vi "ActionVIOnDownload.vi"(5 "System Definition Dir":path, 6 "IP address":string, 7 "Details Ref":refnum<vi>, 8 "error in (no error)":errorcluster, 10 "WebDAV session in":T1, 11 "Device Item Ref in":T2 format="%.0x") -> (0 "error out":errorcluster, 2 "WebDAV session out":T1, 3 "Device Item Ref out":T2 format="%.0x")   [LabVIEW 2020, in "XNET System Explorer.lvlib"]
uses:
  XNET System Explorer.lvlib
  <vilib>/NI VeriStand/Custom Device API/Custom Device Item Ref.ctl
  <vilib>/WebDAVClient/Advanced/SessionHandle.ctl
  Includes/XNET System Explorer.lvlibp/System Explorer/Implementation/Implementation.lvlib
  <vilib>/NI VeriStand/Custom Device API/Custom Device API.lvlib
  <vilib>/WebDAVClient/NI_WebDAV.lvlib
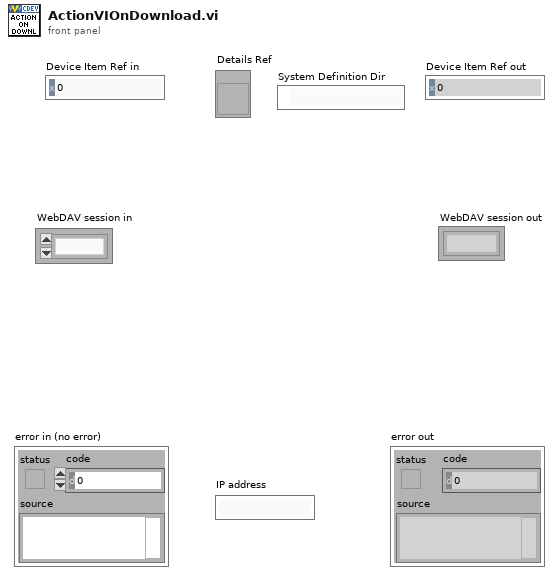
[diagram p1: front panel]
types:
  T1 = typedef "NI_WebDAV.lvlib/SessionHandle.ctl" = refnum<k1>
  T2 = typedef "Custom Device API.lvlib/Custom Device Item Ref.ctl" = u64
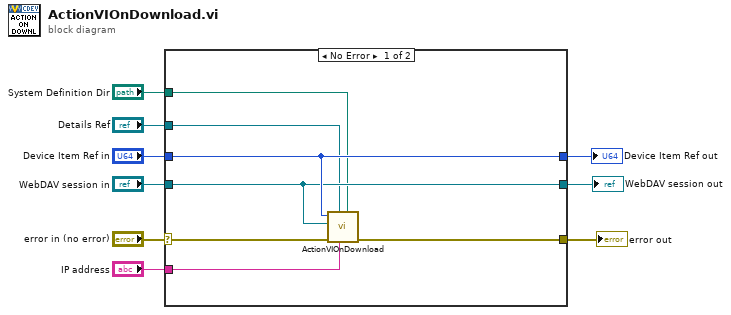
[diagram p0: block diagram]
diagram:
  n1 = case shown="No Error" "error in (no error)" {
    selector: "error in (no error)" -> [w16 w19]
    tunnel: [w15 w19] -> w8
    tunnel: "WebDAV session in" -> [w13 w18]
    tunnel: [w13 w18] -> w4
    tunnel: "Device Item Ref in" -> [w14 w17]
    tunnel: [w14 w17] -> w6
    tunnel: "Details Ref" -> [w12 _]
    tunnel: "IP address" -> [w11 _]
    tunnel: "System Definition Dir" -> [w10 _]
    frame No Error {
      n2 = call "ActionVIOnDownload.vi"("System Definition Dir"=w10, "IP address"=w11, "Details Ref"=w12, "error in (no error)"=w16, "WebDAV session in"=w13, "Device Item Ref in"=w14) -> ("error out"=w15:errorcluster)  [unwired: 3 in, 2 out]
    }
    frame Error {
    }
  }
  "error out" <- w8
  "Device Item Ref out" <- w6
  "WebDAV session out" <- w4
